vi "Tool data gatheringloop.vi"(1 "Loop ID":T1, 11 "error out":errorcluster) -> ()   [LabVIEW 2011]
uses:
  Application Structure/Loop ID.ctl
  Common/Variable List Common Digital.ctl
  Common/Variable List Common Analog.ctl
  Action Analog Handler.ctl
  Tool/Stroker/High level/Variable List Stroker Analog.ctl
  emi Lib/System 01/0 - General/App/Loop control 2/Private/_emi_ SMLoop start condition.vi
  emi Lib/System 01/0 - General/App/Loop control 2/Private/_emi_ SMLoop Error Check.vi
  emi Lib/Basic/0 - General/Error/emi_Is Error.vi
  emi Lib/System 01/0 - General/App/Loop control 2/Private/_emi_SMLoop Register new.vi
  emi Lib/System 01/0 - General/S&E reporting/emi_Send S&E Error message.vi
  emi Lib/Basic/0 - General/Error/emi_ Is Error state.vi
  emi Lib/System 01/0 - General/emi_Read System ID.vi
  emi Lib/System 01/0 - General/App/Loop control/Private/_emi_GFV Loop Linking.vi
  emi Lib/System 01/0 - General/App/Loop control/Private/_emi_GFV Loop Enable.vi
  emi Lib/System 01/0 - General/App/Loop control 2/Private/_emi_ SMLoop Restart.vi
  emi Lib/System 01/0 - General/App/Private/_emi_GFV App Close.vi
  emi Lib/System 01/0 - General/App/Loop control 2/Private/_emi_ SMLoop Restart Counter.vi
  emi Lib/System 01/0 - General/App/Loop control/Private/_emi_GFV Loop Running.vi
  emi Lib/System 01/0 - General/Private/_emi_GFV System ID.vi
  emi Lib/System 01/0 - General/S&E reporting/Private/_emi_S&E Q Generator.vi
  <vilib>/Utility/error.llb/Clear Errors.vi
  emi Lib/System 01/0 - General/App/Loop control/Private/_emi_GFV stop a loop so it can reset.vi
  <vilib>/Utility/VariantDataType/GetNumericInfo.vi
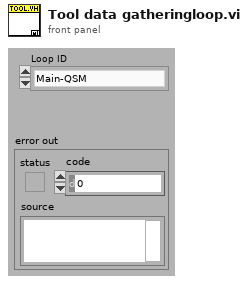
[diagram p1: front panel]
types:
  T1 = typedef "Loop ID.ctl" = enum16{"Main-QSM", "Main-Dialog", "Main-Ind Upd", "Main-Graph Upd", "Main-Debug", "Main-DebugW1", "Main-DebugW2", "Main-SE Handler", "Interface-PCP", "Interface-CANbus", "Interface-Modem", "Var Handling-Beat", "Var Handling-From PCP", "Var Handling-File storage", "Var Handling-From Simulator", "GUI-GrphW Mast", "GUI-GrphW Slav", "SIM-Tool W1", "SIM-Tool W2", "Alm-Sound", "LEIN-motor", "Tool data gatherer Qer", "Tool Data LEIN STAT2 dekoder", "Indicator Value Update", "Tool STAT2 dedicated reader", "Tool ID handler", "Detail View L1", "Detail View L2", "Main display enable view", "Sequence runner", "Voltage setpoint", "Resistance setpoint", "Stroker Wizard L1", "Stroker Wizard L2", "Alarm Handling", "Annotations Tip Strip", "Magna Interface"}
  T2 = typedef "Variable List Common Digital.ctl" = enum16{"PCP Connected", "PCP PC Control", "HV PSU connected", "HV PSU HV Active", "Modem Connected", "Tool Connected", "CanBus interface"}
  T3 = typedef "Variable List Common Analog.ctl" = enum16{"HVPSU Head Voltage", "HVPSU TS Voltage", "HVPSU Current", "PCP Cable Resistance", "Winch Depth", "Winch Line Speed", "Winch Wire Tension"}
  T4 = typedef "Action Analog Handler.ctl" = enum16{"GET value", "GET Single Frequenzy", "GET All Values", "GET Waveform", "Get Numb Var", "SET Value", "START Buffer", "REG Variable", "BUF size(total antal sekund)", "PULS", "Get a Value at time", "Set initial waveform"}
  T5 = typedef "Variable List Stroker Analog.ctl" = enum16{"Tool max Temperature", "Solenoid Temp", "Tool supply Voltage", "Tool (Controller) Current", "Tool Acceleration X", "Tool Acceleration Y", "Tool Acceleration Z", "Controller Temp", "Tool Acceleration Sum", "Tool Inclination", "Tool Rotation", "Tool Stroke Extension", "Tool GP Sensor 1", "Tool GP Sensor 2", "Tool (Pressure 1) Temp", "Tool Pressure 1", "Tool (Pressure 2) Temp", "Tool Pressure 2", "Do not use (SIF)", "Do not use (SOF)", "Stroke Force", "PSU Temp", "Head Voltage", "PSU Main Voltage out", "PSU Main Current out", "Upper Tension Sub Temp", "Tool Upper Tension Sub", "Lower Tension Sub Temp", "Tool Lower Tension Sub"}
  T6 = typedef "_emi_ SMLoop sates.ctl" = enum16{"Init", "Standby", "Start", "Normal Operation", "Stop", "Error Handling", "End", "Post"}
  T7 = cluster{"Placeholder":bool, "Tool Data not":refnum<notifier>, "Ana com":i32, "Dig com":i32}
  T8 = typedef "Options  All pages and custom.ctl" = cluster{"P 1 (App)":T9, "P 2":T10, "P 3":T11, "P 4":T14, "P 5":T18, "P 6 (Err)":T19, "P 7 (Expert)":T20, "C 1":T22, "C 2":T24}
  T9 = typedef "Options Page 1 (App).ctl" = cluster{"Result files":path, "PCP Interface":string, "Tractor/Stroker Interface":string, "Tractor Interface":string, "Audible Alarm":bool, "Force alarm on Technical":bool, "Force alarm on HH":bool, "Force alarm on LL":bool, "Force alarm on H":bool, "Force alarm on L":bool}
  T10 = typedef "Options Page 2.ctl" = cluster{"Solenoid & Relay latching time":u16, "Tractor relay 1":dbl, "Tractor relay 2":dbl, "Tractor Solenoid limit":dbl}
  T11 = typedef "Options Page 3.ctl" = cluster{"Min resistance":dbl, "Max resistance":dbl, "PCP/PSU range":T12, "Max voltage jump":dbl, "Maximum resistance change":dbl, "Start Telemetry Voltage":dbl, "Start Telemetry Timeout":dbl, "Start Motor Voltage":dbl, "Stop Motor Voltage":dbl, "Pass Mode Warning Voltage":dbl, "Relay Switch Voltage":dbl, "Winch Spool Circumference":dbl, "Winch Pulses per Revolution":dbl, "Samples to average":i32, "PSU type":T13, "Magna OVP":dbl, "Magna Current Limit":dbl}
  T12 = typedef "PCP type List.ctl" = enum16{"0 - 350V", "0 - 450V", "0 - 600V"}
  T13 = typedef "PSU Type.ctl" = enum16{"Unipower", "Magna"}
  T14 = typedef "Options Page 4.ctl" = cluster{"Solenoid & Relay latching time":u16, "Stroker relay 1":dbl, "Stroker Relay 2":dbl, "Stroker Solenoid limit":dbl, "Force det.":T15, "Stroke force lim.":dbl, "Pressure SLIPS":dbl, "Tacometer puls":dbl, "Default anchor behavior":T16, "Default stroker behavior":T17, "Default stroker force limit (tonne)":dbl}
  T15 = typedef "Stroke force selector.ctl" = enum16{"Stroke in = node 1", "Strok out = node 1"}
  T16 = typedef "Default anchor behavior.ctl" = enum16{"Do nothing", "Set Anchor", "Release Anchor"}
  T17 = typedef "Default stroker behavior.ctl" = enum16{"Do nothing", "Stop", "Go Out", "Go In"}
  T18 = typedef "Options Page 5.ctl" = cluster{"Solenoid & Relay latching time":u16, "Driller relay 1":dbl, "Driller Relay 2":dbl, "Driller  Solenoid limit":dbl}
  T19 = typedef "Options Page 6 (Err).ctl" = cluster{"Error and event files":path}
  T20 = typedef "Options Page 7 (Expert).ctl" = cluster{"Show Debug":bool, "Log debug messages":bool, "Additional debug messages":bool, "Start Beagle with Simulator data":bool, "Workshop mode":bool, "Modem baud":u16, "enumCANCOM":bool, "Modem sim":T21, "Telemetry Timeout Disable":i32, "Buffer size":i32, "Upd regular data":bool}
  T21 = typedef "Modem simulation setup.ctl" = cluster{"Modem dealay sim":bool, "Sim baud Tx":u16, "Bit Error fraction Tx":dbl, "Sim baud Rx":u16, "Bit Error fraction Rx":dbl}
  T22 = typedef "Options Custom 1.ctl" = cluster{"Placeholder":bool, "Slips Size":T23}
  T23 = typedef "Slips Type Radio.ctl" = enum32{"No Selection", "338 MRS", "3,9 MRS"}
  T24 = typedef "Options Custom 2.ctl" = cluster{"Placeholder":bool}
  T25 = typedef "Fixed Analog Channel Definition.ctl" = cluster{"ID":u16, "Name":string, "Quantity":T26, "Unit":string, "Maximum upd":T27, "Comment":string, "Help file Name":string, "Help file Section ":string, "Category":T28, "User adjustable Scaling":bool, "Default Scaling":T29, "In use":bool, "Default Unit":i32}
  T26 = typedef "Quantity enum.ctl" = enum16{"Acceleration", "Angle", "Current", "Force", "Distance", "Pressure", "Resistance", "Rotational Speed", "Speed", "Temperature", "Tension", "Torque", "Voltage", "Weight"}
  T27 = typedef "Update frequensies.ctl" = enum16{"2 Hz", "1 Hz", "0.1 Hz"}
  T28 = typedef "Channel catagory Enum.ctl" = enum16{"No Category", "Power", "Temperature", "Pressure"}
  T29 = typedef "Scaling.ctl" = cluster{"Gain":dbl, "Offset":dbl}
  T30 = typedef "Fixed Digital Channel Definition.ctl" = cluster{"ID":u16, "Name":string, "NA Text":string, "Off Text":string, "On Text":string, "Maximum upd":T27, "Comment":string, "Help file Name":string, "Help file Section ":string, "Catagory":T28, "In use":bool}
  T31 = typedef "Tool simulator data.ctl" = cluster{"Analog Values":dbl[], "Digital Values":T32[]}
  T32 = typedef "Status Digitalish.ctl" = enum16{"NA", "False", "True"}
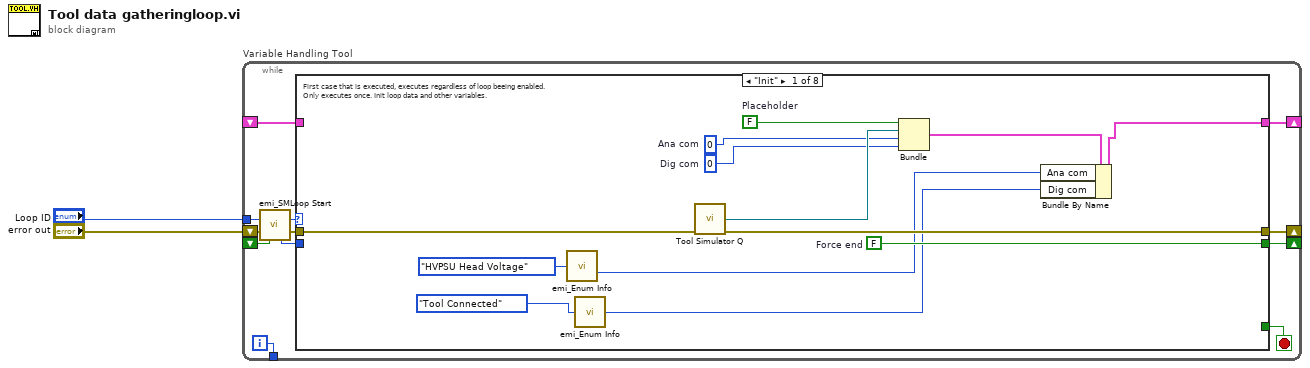
[diagram p0: block diagram]
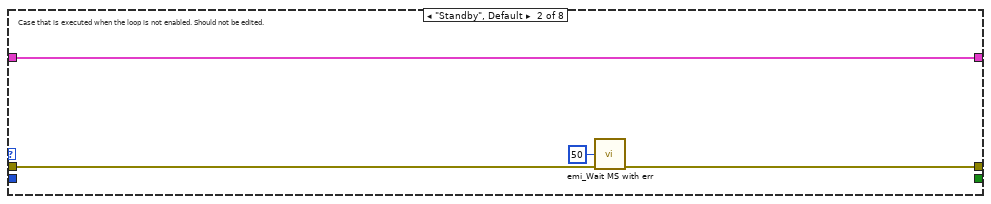
[diagram p2: hidden frame]
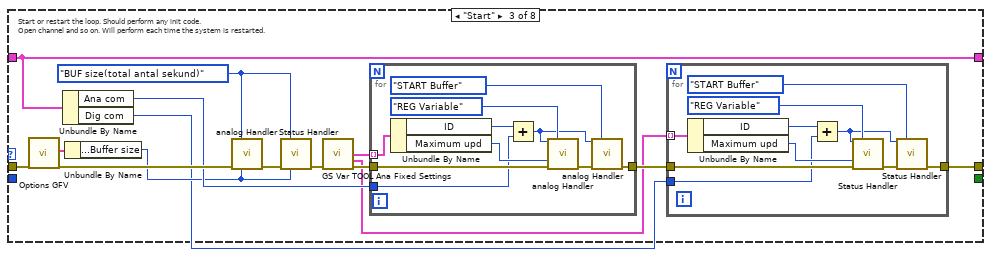
[diagram p3: hidden frame]
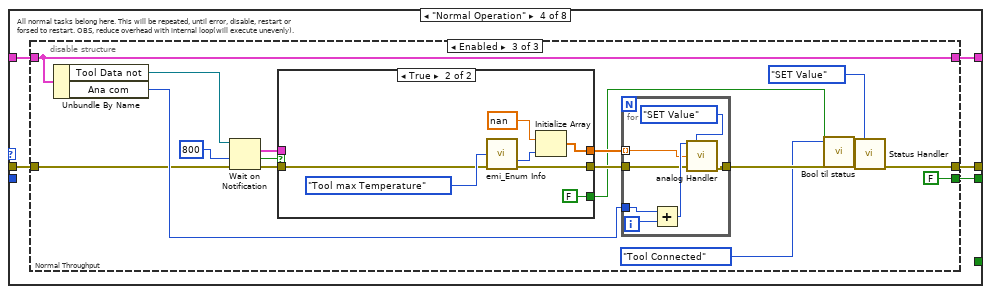
[diagram p4: hidden frame]
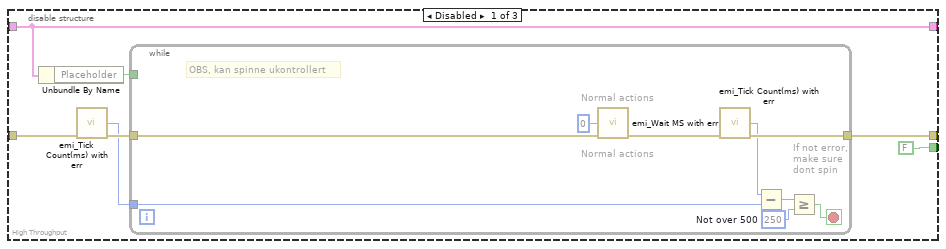
[diagram p5: hidden frame]
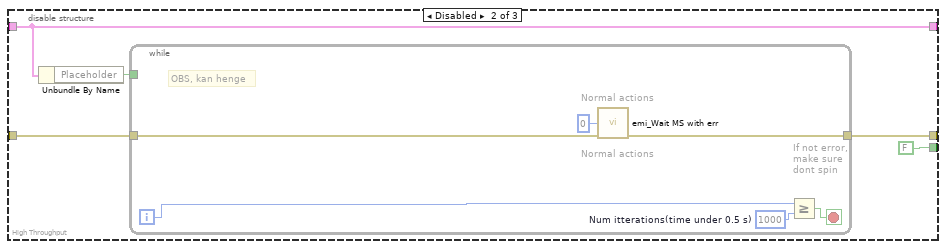
[diagram p6: hidden frame]
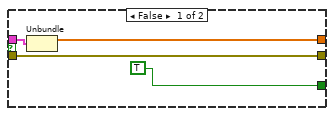
[diagram p7: hidden frame]
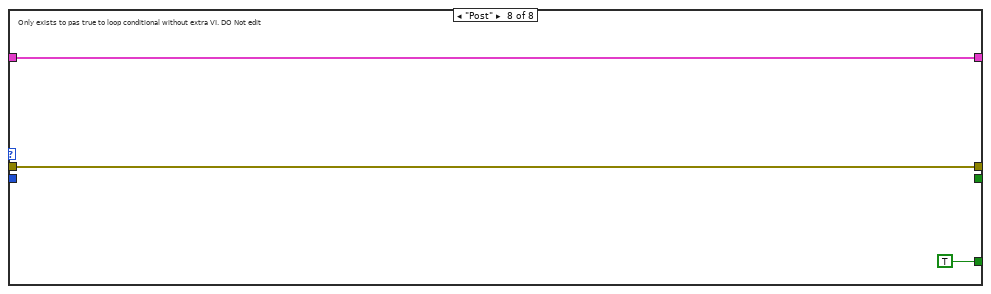
[diagram p11: hidden frame]
diagram:
  n1 = while "Variable Handling Tool" {
    shift-right: [w14] -> _
    shift-left: _ -> [w10]
    shift-right: [w12] -> _
    shift-left: "error out" -> [w8]
    tunnel: [w11] -> _
    shift-right: [w9] -> _
    shift-left: _ -> [w4]
    tunnel: "Loop ID" -> [w5]
    i -> [w11]
    stop <- w13 stop-if-true
    n2 = call "emi_SMLoop Start.vi"("Loop ID"=w5, "error in (no error)"=w8, "Force Stop(F)"=w4) -> ("Loop command"=w6:T6, "error out"=w7:errorcluster, "Loop ID out"=w3:i32)  [unwired: 10 in]
    n3 = case shown="\"Init\"" w6 {
      tunnel: [w19 w28 w41 w69 w134 w137 w138 w141] -> w14
      tunnel: [_ _ _ _ _ _ _ TRUE] -> w13
      tunnel: w7 -> [w24 w30 w42 w71 w135 w136 w139 w142]
      tunnel: [w23 w29 w35 w70 w135 w136 w139 w142] -> w12
      tunnel: w10 -> [_ w28 w41 w68 w134 w137 w138 w141]
      tunnel: [w25 _ _ w67 _ _ _ _] -> w9
      tunnel: w3 -> [_ _ _ _ _ _ _ _]
      frame "Init" {
        w17 = 0  # Dig com
        w18 = 0  # Ana com
        w25 = FALSE  # Force end
        w26 = FALSE  # Placeholder
        # "First case that is executed, executes regardless of loop beeing enabled.\nOnly executes once. Init loop data and other variables."
        n4 = call "emi_Enum Info.vi"("Enum"=Variable_List_Common_Analog."HVPSU Head Voltage" ("Action")) -> ("Numb Elements"=w16:i32)  [unwired: 11 in, 3 out]
        n5 = call "emi_Enum Info.vi"("Enum"=Variable_List_Common_Digital."Tool Connected" ("Action")) -> ("Numeric Value"=w15:u64)  [unwired: 11 in, 3 out]
        n6 = call "Tool Simulator Q.vi"("error in (no error)"=w24) -> ("Tool Data not"=w22:refnum<notifier>, "error out"=w23:errorcluster)  [unwired: 12 in, 1 out]
        n7 = Bundle("Placeholder"=w26, "Tool Data not"=w22, "Ana com"=w18, "Dig com"=w17) -> (w27:T7)  [unwired: 1 in]
        n8 = Bundle By Name(cluster=w27, "Ana com"=w16, "Dig com"=w15) -> (w19:T7)
      }
      frame "Standby", Default {
        # "Case that is executed when the loop is not enabled. Should not be edited."
        n9 = call "emi_Wait MS with err.vi"("milliseconds to wait(0)"=u32 50, "error in (no error)"=w30) -> ("error out"=w29:errorcluster)  [unwired: 13 in]
      }
      frame "Start" {
        w38 = Action_Analog_Handler."BUF size(total antal sekund)" ("Action(GET)")
        # "Start or restart the loop. Should perform any init code. \nOpen channel and so on. Will perform each time the system is restarted."
        n10 = call "Options GFV.vi"("error in (no error)"=w42) -> ("Options"=w45:T8, "error out"=w46:errorcluster)  [unwired: 16 in, 1 out]
        n11 = Unbundle By Name(w41) -> ("Ana com"=w40:i32, "Dig com"=w32:i32)
        n12 = Unbundle By Name(w45) -> ("P 7 (Expert).Buffer size"=w37:i32)
        n13 = call "analog Handler.vi"("Action"=w38, "error in (no error)"=w46, "Start tid / buf size"=w37) -> ("error out"=w39:errorcluster)  [unwired: 7 in, 5 out]
        n14 = call "Status Handler.vi"("Action"=w38, "error in (no error)"=w39, "Start tid(buff size"=w37) -> ("error out"=w34:errorcluster)  [unwired: 8 in, 4 out]
        n15 = call "GS Var TOOL Ana Fixed Settings.vi"("error in (no error)"=w34) -> ("Tool Analog var Fixed out"=w43:T25[], "Tool Digital Var Fixed out"=w33:T30[], "error out"=w44:errorcluster)  [unwired: 12 in]
        n16 = for {
          tunnel: [w61] -> w36
          tunnel: w44 -> [w66]
          tunnel: w43 -> [w65] mode=indexing
          tunnel: w40 -> [w57]
          n17 = Unbundle By Name(w65) -> ("ID"=w60:u16, "Maximum upd"=w64:T27)
          n18 = Add(x=w60, y=w57) -> (x+y=w58:i32)
          n19 = call "analog Handler.vi"("Variable Index"=w58, "Action"=Action_Analog_Handler."REG Variable" ("Action(GET)"), "Upd freq"=w64, "error in (no error)"=w66) -> ("error out"=w62:errorcluster)  [unwired: 6 in, 5 out]
          n20 = call "analog Handler.vi"("Variable Index"=w58, "Action"=Action_Analog_Handler."START Buffer" ("Action(GET)"), "error in (no error)"=w62) -> ("error out"=w61:errorcluster)  [unwired: 7 in, 5 out]
        }
        n21 = for {
          tunnel: [w51] -> w35
          tunnel: w36 -> [w56]
          tunnel: w33 -> [w55] mode=indexing
          tunnel: w32 -> [w47]
          n22 = Unbundle By Name(w55) -> ("ID"=w50:u16, "Maximum upd"=w54:T27)
          n23 = Add(x=w50, y=w47) -> (x+y=w48:i32)
          n24 = call "Status Handler.vi"("Variable Index"=w48, "Action"=Action_Analog_Handler."REG Variable" ("Action(GET)"), "Upd freq"=w54, "error in (no error)"=w56) -> ("error out"=w52:errorcluster)  [unwired: 7 in, 4 out]
          n25 = call "Status Handler.vi"("Variable Index"=w48, "Action"=Action_Analog_Handler."START Buffer" ("Action(GET)"), "error in (no error)"=w52) -> ("error out"=w51:errorcluster)  [unwired: 8 in, 4 out]
        }
      }
      frame "Normal Operation" {
        # "All normal tasks belong here. This will be repeated, until error, disable, restart or\nforsed to restart. OBS, reduce overhead with internal loop(will execute unevenly)."
        n26 = disable-structure shown="Enabled" {
          disable-tunnel: w71 -> [w75 w88 w105]
          disable-tunnel: [w77 w91 w102] -> w70
          disable-tunnel: [w78 w92 w112] -> w69
          disable-tunnel: w68 -> [w78 w92 w112]
          disable-tunnel: [FALSE ("Force End") FALSE ("Force End") FALSE ("Force End")] -> w67
          frame Disabled {
            # "High Throughput"
            n27 = Unbundle By Name(w78) -> ("Placeholder"=w76:bool)
            n28 = call "emi_Tick Count(ms) with err.vi"("error in (no error)"=w75) -> ("millisecond timer value"=w73:u32, "error out"=w74:errorcluster)  [unwired: 13 in]
            n29 = while {
              tunnel: w74 -> [w81]
              tunnel: [w87] -> w77
              tunnel: w76 -> [_]
              tunnel: w73 -> [w86]
              stop <- w80 stop-if-true
              w83 = u32 250  # Not over 500
              # "OBS, kan spinne ukontrollert"
              # "If not error,\nmake sure \ndont spin"
              # "Normal actions"
              # "Normal actions"
              n30 = call "emi_Wait MS with err.vi"("milliseconds to wait(0)"=u32 0, "error in (no error)"=w81) -> ("error out"=w82:errorcluster)  [unwired: 13 in]
              n31 = call "emi_Tick Count(ms) with err.vi"("error in (no error)"=w82) -> ("millisecond timer value"=w85:u32, "error out"=w87:errorcluster)  [unwired: 13 in]
              n32 = Subtract(x=w85, y=w86) -> (x-y=w84:u32)
              n33 = Greater Or Equal?(x=w84, y=w83) -> (x >= y?=w80:bool)
            }
          }
          frame Disabled {
            # "High Throughput"
            n34 = Unbundle By Name(w92) -> ("Placeholder"=w90:bool)
            n35 = while {
              tunnel: [w94] -> w91
              tunnel: w90 -> [_]
              tunnel: w88 -> [w95]
              i -> [w93]
              stop <- w97 stop-if-true
              w98 = u32 1000  # Num itterations(time under 0.5 s)
              # "OBS, kan henge"
              # "If not error,\nmake sure \ndont spin"
              # "Normal actions"
              # "Normal actions"
              n36 = call "emi_Wait MS with err.vi"("milliseconds to wait(0)"=u32 0, "error in (no error)"=w95) -> ("error out"=w94:errorcluster)  [unwired: 13 in]
              n37 = Greater Or Equal?(x=w93, y=w98) -> (x >= y?=w97:bool)
            }
          }
          frame Enabled {
            # "Normal Throughput"
            n38 = Unbundle By Name(w112) -> ("Tool Data not"=w113:refnum<notifier>, "Ana com"=w106:i32)
            n39 = Wait on Notification(notifier=w113, timeout in ms (-1)=800, error in (no error)=w105) -> (notification=w109:T31, timed out?=w110:bool, error out=w111:errorcluster)  [unwired: 1 in, 1 out]
            n40 = case shown="True" w110 {
              tunnel: w111 -> [w124 w132]
              tunnel: w109 -> [w126 _]
              tunnel: [w125 w129] -> w108
              tunnel: [w124 w128] -> w107
              tunnel: [TRUE ("Tool") FALSE ("Tool")] -> w99
              frame False {
                n41 = Unbundle(w126) -> ("Analog Values"=w125:dbl[])  [unwired: 1 out]
              }
              frame True {
                n42 = call "emi_Enum Info.vi"("Enum"=Variable_List_Stroker_Analog."Tool max Temperature" ("Action"), "error in (no error)"=w132) -> ("Numb Elements"=w131:i32, "error out"=w128:errorcluster)  [unwired: 10 in, 2 out]
                n43 = Initialize Array(nan ("element"), w131) -> (w129:dbl[])
              }
            }
            n44 = for {
              tunnel: w108 -> [w119] mode=indexing
              tunnel: w107 -> [w118]
              tunnel: [w117] -> w103
              tunnel: w106 -> [w116]
              i -> [w122]
              n45 = Add(x=w116, y=w122) -> (x+y=w120:i32)
              n46 = call "analog Handler.vi"("Variable Index"=w120, "Action"=Action_Analog_Handler."SET Value" ("Action(GET)"), "Value"=w119, "error in (no error)"=w118) -> ("error out"=w117:errorcluster)  [unwired: 6 in, 5 out]
            }
            n47 = call "Bool til status.vi"("Boolean"=w99) -> ("Status"=w104:T32)  [unwired: 8 in]
            n48 = call "Status Handler.vi"("Variable Index"=Variable_List_Common_Digital."Tool Connected" ("Action"), "Action"=Action_Analog_Handler."SET Value", "Value"=w104, "error in (no error)"=w103) -> ("error out"=w102:errorcluster)  [unwired: 7 in, 4 out]
          }
        }
      }
      frame "Stop" {
        # "Stop the loop. May be restarted later. Close interfaces and the like"
      }
      frame "Error Handling" {
        # "Loop automaticaly returns here after error is found. If error is cleared, \nLoop wil continue as normal(if was operative when error."
      }
      frame "End" {
        # "Only executes at application end has. Should performa any action the loop \nneeds to finnish. Executes only once."
      }
      frame "Post" {
        # "Only exists to pas true to loop conditional without extra VI. DO Not edit"
      }
    }
  }
